vi "Post-Build Action.vi"(5 "Files Generated by Build":path[](array[path]), 6 "Top Level/Always Included VIs":path[](array[path]), 7 "Destination Path":path, 8 "error in (no error)":errorcluster, 9 "Target Name":string, 10 "Build Specification Name":string, 11 "Project Path":path) -> (0 "error out":errorcluster)   [LabVIEW 2020, in "Build Support.lvlib"]
uses:
  Build Support.lvlib
  <vilib>/Utility/miscctls.llb/LVReplaceWithSaveOptionEnum.ctl
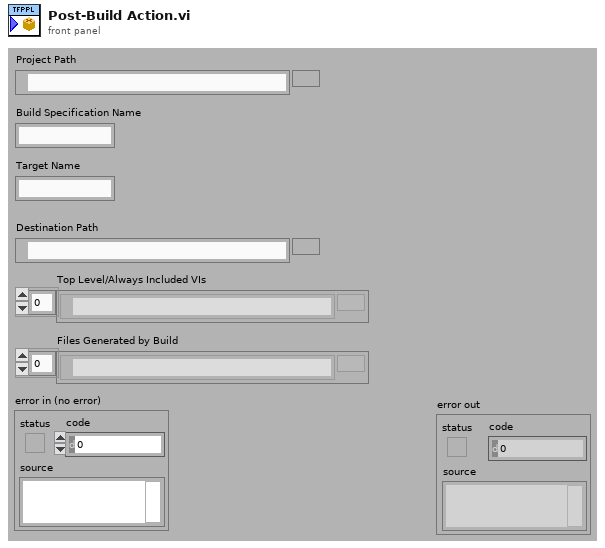
[diagram p1: front panel]
types:
  T1 = typedef "LVReplaceWithSaveOptionEnum.ctl" = enum16{"Save All Without Prompts", "Save All With Prompts", "Do Not Save (Retain In Memory)"}
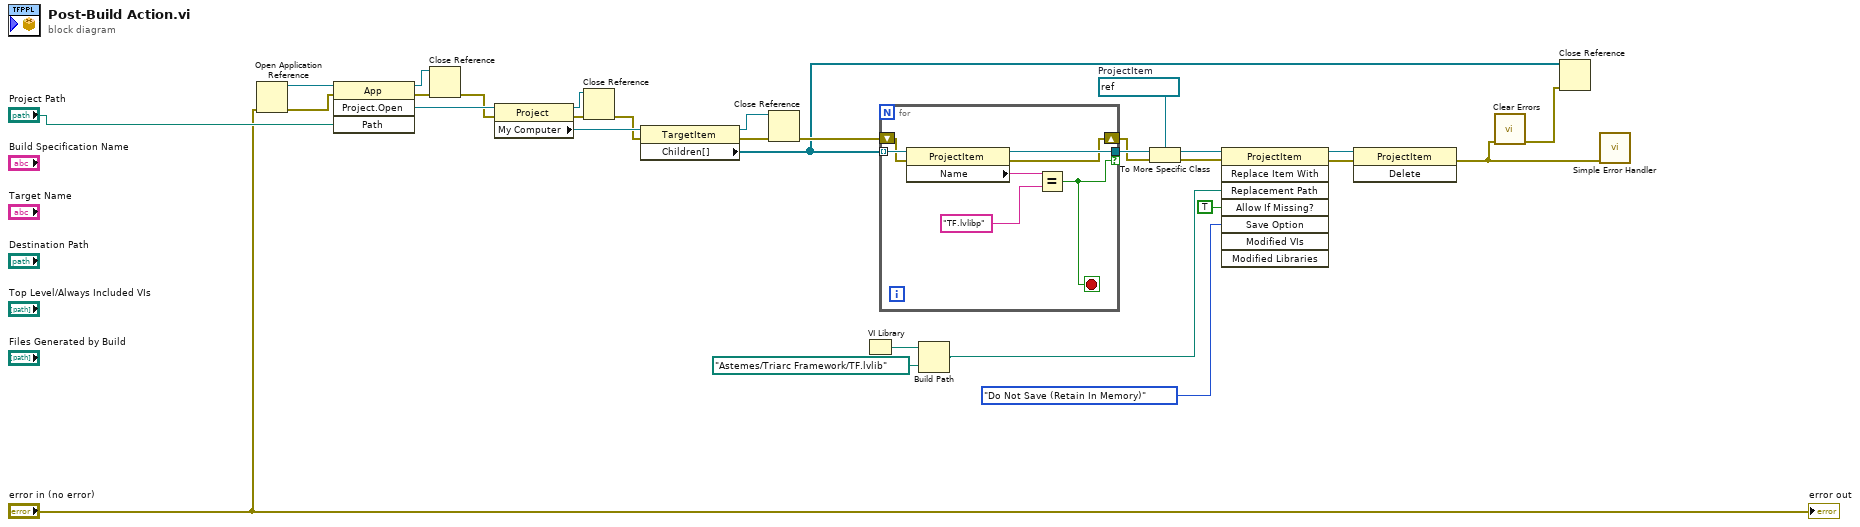
[diagram p0: block diagram]
diagram:
  w16 = refnum<vi> refnum  # ProjectItem
  n1 = Open Application Reference(8:"error in (no error)") -> (0:w29:errorcluster, 3:w30:refnum<vi>)  [unwired: 3 in]
  n2 = invoke class="App" method="Project.Open"(reference=w30, error in=w29, "Path"="Project Path") -> (reference out=w22:refnum<vi>, error out=w26:errorcluster, "Project:Open"=w28:refnum<vi>)  [unwired: 1 in, 1 out]
  n3 = Close Reference(reference=w22, error in (no error)=w26) -> (error out=w23:errorcluster)
  n4 = property class="Project"(reference=w28, error in=w23) -> (reference out=w20:refnum<vi>, error out=w25:errorcluster, "My Computer"=w27:refnum<vi>)
  n5 = Close Reference(reference=w20, error in (no error)=w25) -> (error out=w21:errorcluster)
  n6 = property class="TargetItem"(reference=w27, error in=w21) -> (reference out=w19:refnum<vi>, error out=w24:errorcluster, "Children[]"=w6:refnum<vi>[])
  n7 = Close Reference(reference=w19, error in (no error)=w24) -> (error out=w10:errorcluster)
  n8 = VI Library() -> (path=w9:path)
  n9 = for {
    tunnel: w6 -> [w37] mode=indexing
    tunnel: [w34] -> w17 if=w33
    shift-right: [w31] -> w12
    shift-left: w10 -> [w32]
    stop <- w33 stop-if-true
    n10 = property class="ProjectItem"(reference=w37, error in=w32) -> (reference out=w34:refnum<vi>, error out=w31:errorcluster, "Name"=w36:string)
    n11 = Equal?(x=w36, y="TF.lvlibp") -> (x = y?=w33:bool)
  }
  n12 = Build Path(base path=w9, name or relative path=path "Astemes/Triarc Framework/TF.lvlib") -> (appended path=w7:path)
  n13 = To More Specific Class(target class=w16, reference=w17, error in=w12) -> (specific class reference=w15:refnum<vi>, error out=w11:errorcluster)
  n14 = invoke class="ProjectItem" method="Replace Item With"(reference=w15, error in=w11, "Replacement Path"=w7, "Allow If Missing?"=TRUE, "Save Option"=LVReplaceWithSaveOptionEnum."Do Not Save (Retain In Memory)") -> (reference out=w1:refnum<vi>, error out=w3:errorcluster)  [unwired: 3 in, 6 out]
  n15 = invoke class="ProjectItem" method="Delete"(reference=w1, error in=w3) -> (error out=w2:errorcluster)  [unwired: 1 in, 2 out]
  n16 = call <vilib>:"Clear Errors.vi"("error in (no error)"=w2) -> ("error out"=w5:errorcluster)  [unwired: 5 in, 1 out]
  n17 = Close Reference(reference=w6, error in (no error)=w5) -> ()  [unwired: 1 out]
  n18 = call <vilib>:"Simple Error Handler.vi"("error in (no error)"=w2) -> ()  [unwired: 4 in, 5 out]
  "error out" <- "error in (no error)"
